vi "Destroy Events.vi"(8 "error in":errorcluster, 11 "Events":T1) -> (0 "error out":errorcluster)   [LabVIEW 2020, in "Counter.lvlib"]
uses:
  Counter.lvlib
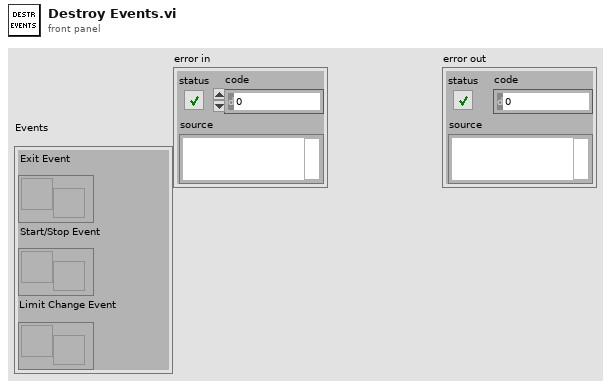
[diagram p1: front panel]
types:
  T1 = cluster{"Exit Event":refnum<user-event>, "Start/Stop Event":refnum<user-event>, "Limit Change Event":refnum<user-event>}
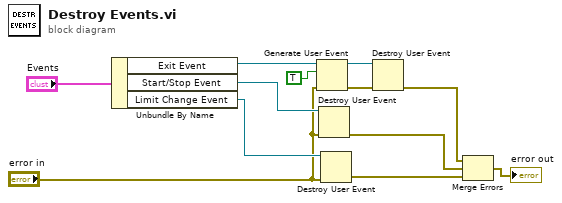
[diagram p0: block diagram]
diagram:
  n1 = Unbundle By Name("Events") -> ("Exit Event"=w11:refnum<user-event>, "Start/Stop Event"=w8:refnum<user-event>, "Limit Change Event"=w7:refnum<user-event>)
  n2 = Generate User Event(user event=w11, event data cluster=TRUE ("event data"), error in="error in") -> (user event out=w9:refnum<user-event>, error out=w10:errorcluster)  [unwired: 1 in]
  n3 = Destroy User Event(user event=w8, error in="error in") -> (error out=w3:errorcluster)
  n4 = Destroy User Event(user event=w7, error in="error in") -> (error out=w2:errorcluster)
  n5 = Destroy User Event(user event=w9, error in=w10) -> (error out=w5:errorcluster)
  n6 = Merge Errors(w5, w3, w2) -> (→"error out":errorcluster)
